vi "Obtain Request Events.vi"(8 "error in (no error)":errorcluster, 10 "Create New?":bool) -> (0 "error out":errorcluster, 2 "Device Under Test_Cloneable_DQMH Request Events":T1)   [LabVIEW 2015, in "Device Under Test_Cloneable_DQMH.lvlib"]
doc: "This VI Obtains/Creates the Requests events that will be used for other modules to communicate with the module that owns this VI. These Requests events will be accessed only via Public API methods for this module.\n\n<b>NOTE</b>: The contents of this VI are automatically generated and modified by the <b>Tools > Delacor > DQMH</b> utilities. Consider using those utilities instead of making your own modifications to this VI.\n_____\nBased on Delacor QMH Project Template 2.0.0.62.\n____\nDelacor QMH Thermal Chamber Examples 4.0.0.21\nCopyright (c) 2018, Delacor"
uses:
  Device Under Test_Cloneable_DQMH.lvlib
  Request Events--cluster.ctl
  Stop Argument--cluster.ctl
  Show Panel Argument--cluster.ctl
  Hide Panel Argument--cluster.ctl
  Show Diagram Argument--cluster.ctl
  Set Power State Argument--cluster.ctl
  Perform Self Test Argument--cluster.ctl
  Perform Self Test (Reply Payload)--cluster.ctl
  Update DUT Status Argument--cluster.ctl
  Get Module Execution Status Argument--cluster.ctl
panel:
  # "NOTE: The contents of this VI are automatically generated and modified by the Tools > Delacor > DQMH utilities. Consider using those utilities instead of making your own modifications to this VI."
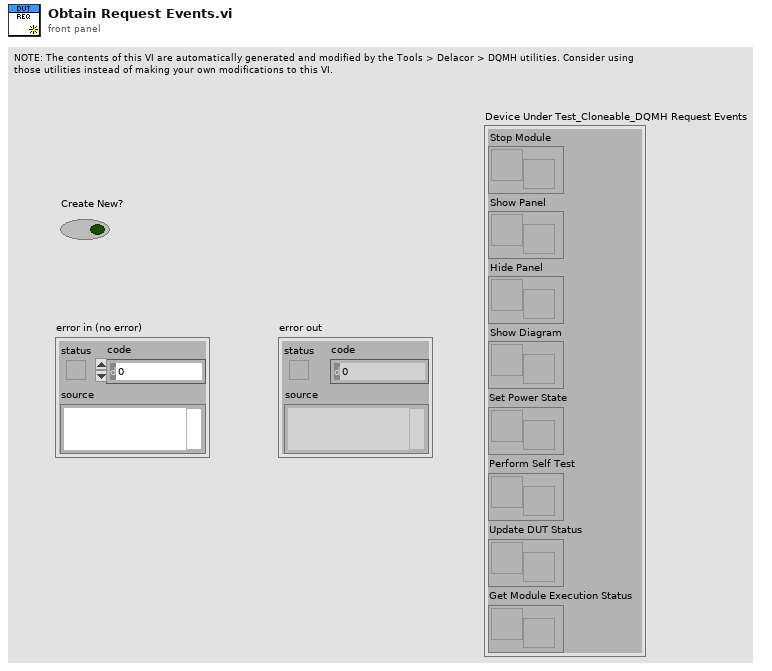
[diagram p1: front panel]
types:
  T1 = typedef "Device Under Test_Cloneable_DQMH.lvlib/Request Events--cluster.ctl" = cluster{"Stop Module":refnum<user-event>, "Show Panel":refnum<user-event>, "Hide Panel":refnum<user-event>, "Show Diagram":refnum<user-event>, "Set Power State":refnum<user-event>, "Perform Self Test":refnum<user-event>, "Update DUT Status":refnum<user-event>, "Get Module Execution Status":refnum<user-event>}
  T2 = typedef "Device Under Test_Cloneable_DQMH.lvlib/Get Module Execution Status Argument--cluster.ctl" = cluster{"Module ID":i32, "Running?":bool}
  T3 = typedef "Device Under Test_Cloneable_DQMH.lvlib/Update DUT Status Argument--cluster.ctl" = cluster{"Module ID":i32, "Self Test Result":bool, "Power State":bool}
  T4 = typedef "Device Under Test_Cloneable_DQMH.lvlib/Perform Self Test Argument--cluster.ctl" = cluster{"Module ID":i32, "Wait Notifier":refnum<notifier>}
  T5 = typedef "Device Under Test_Cloneable_DQMH.lvlib/Set Power State Argument--cluster.ctl" = cluster{"Module ID":i32, "Power State":bool}
  T6 = typedef "Device Under Test_Cloneable_DQMH.lvlib/Show Diagram Argument--cluster.ctl" = cluster{"Module ID":i32, "Debug?":bool}
  T7 = typedef "Device Under Test_Cloneable_DQMH.lvlib/Show Panel Argument--cluster.ctl" = cluster{"Show Panel?":bool, "Module ID":i32}
  T8 = typedef "Device Under Test_Cloneable_DQMH.lvlib/Hide Panel Argument--cluster.ctl" = cluster{"Hide Panel?":bool, "Module ID":i32}
  T9 = typedef "Device Under Test_Cloneable_DQMH.lvlib/Stop Argument--cluster.ctl" = cluster{"Origin":string, "Module ID":i32, "Exit via Stop Module Req?":bool, "Wait for Module to stop?":bool}
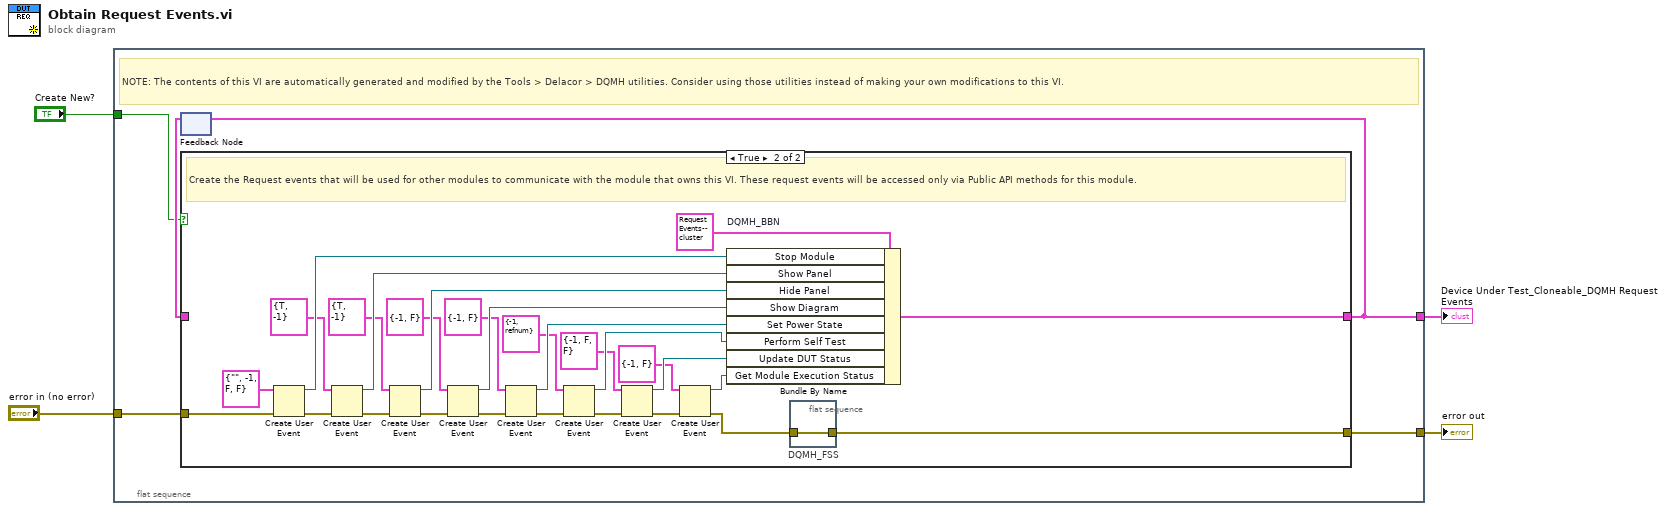
[diagram p0: block diagram]
diagram:
  n1 = flat-sequence {
    tunnel: [w9] -> w4
    tunnel: "error in (no error)" -> [w8]
    tunnel: [w6] -> w2
    tunnel: "Create New?" -> [w5]
    frame #0 {
      # "NOTE: The contents of this VI are automatically generated and modified by the Tools > Delacor > DQMH utilities. Consider using those utilities instead of making your own modifications to this VI."
      n2 = feedback #1() -> (w7:T1)  [unwired: 1 in]
      n3 = case shown="True" w5 {
        tunnel: [w10 w27] -> w9
        tunnel: w8 -> [w10 w39]
        tunnel: [w11 w36] -> w6
        tunnel: w7 -> [w11 _]
        frame False {
        }
        frame True {
          # "Create the Request events that will be used for other modules to communicate with the module that owns this VI. These request events will be accessed only via Public API methods for this module."
          n4 = Create User Event(user event datatype=T9 {"Origin"="", "Module ID"=-1, "Exit via Stop Module Req?"=FALSE, "Wait for Module to stop?"=FALSE} ("Stop Argument"), error in=w39) -> (user event=w37:refnum<user-event>, error out=w34:errorcluster)
          n5 = Create User Event(user event datatype=T7 {"Show Panel?"=TRUE, "Module ID"=-1} ("Show Panel Argument"), error in=w34) -> (user event=w33:refnum<user-event>, error out=w31:errorcluster)
          n6 = Create User Event(user event datatype=T8 {"Hide Panel?"=TRUE, "Module ID"=-1} ("Hide Panel"), error in=w31) -> (user event=w30:refnum<user-event>, error out=w29:errorcluster)
          n7 = Create User Event(user event datatype=T6 {"Module ID"=-1, "Debug?"=FALSE} ("Show Diagram Argument"), error in=w29) -> (user event=w25:refnum<user-event>, error out=w26:errorcluster)
          n8 = Create User Event(user event datatype=T5 {"Module ID"=-1, "Power State"=FALSE} ("Set Power State Argument"), error in=w26) -> (user event=w22:refnum<user-event>, error out=w23:errorcluster)
          n9 = Create User Event(user event datatype=T4 {"Module ID"=-1, "Wait Notifier"=refnum} ("Perform Self Test Argument"), error in=w23) -> (user event=w19:refnum<user-event>, error out=w20:errorcluster)
          n10 = Create User Event(user event datatype=T3 {"Module ID"=-1, "Self Test Result"=FALSE, "Power State"=FALSE} ("Update DUT Status Request Argument"), error in=w20) -> (user event=w16:refnum<user-event>, error out=w17:errorcluster)
          n11 = Create User Event(user event datatype=T2 {"Module ID"=-1, "Running?"=FALSE} ("Get Module Execution Status Argument"), error in=w17) -> (user event=w13:refnum<user-event>, error out=w14:errorcluster)
          n12 = Bundle By Name "DQMH_BBN"(cluster=T1 {"Stop Module"=refnum, "Show Panel"=refnum, "Hide Panel"=refnum, "Show Diagram"=refnum, "Set Power State"=refnum, "Perform Self Test"=refnum, "Update DUT Status"=refnum, "Get Module Execution Status"=refnum} ("output cluster"), "Stop Module"=w37, "Show Panel"=w33, "Hide Panel"=w30, "Show Diagram"=w25, "Set Power State"=w22, "Perform Self Test"=w19, "Update DUT Status"=w16, "Get Module Execution Status"=w13) -> (w36:T1)
          n13 = flat-sequence "DQMH_FSS" {
            tunnel: w14 -> [w40]
            tunnel: [w40] -> w27
            frame #0 {
            }
          }
        }
      }
      n14 = feedback-in #1(w6) -> ()
    }
  }
  "Device Under Test_Cloneable_DQMH Request Events" <- w2
  "error out" <- w4
